vi "Get Buffer Data from Variant.vi"(8 "error in (no error)":errorcluster, 10 "tag":string, 11 "Application Data In in":T2) -> (0 "error out":errorcluster, 1 "Buffer data":T1 {"avg bandwidth" format="%.0g bytes"}, 3 "Application Data In out":T2)   [LabVIEW 2017, in "DSF Core.lvlib"]
uses:
  DSF Core.lvlib
  Main VI/Application Data.ctl
  <vilib>/NI/Memory Manager/Classes/Pointer/Pointer.lvclass
  Classes/Framework/Framework.lvclass
  Buffer Reader/Buffer Data.ctl
  Classes/Buffer/Buffer.lvclass
  Classes/Transfer Group Status/Transfer Group Status.lvclass
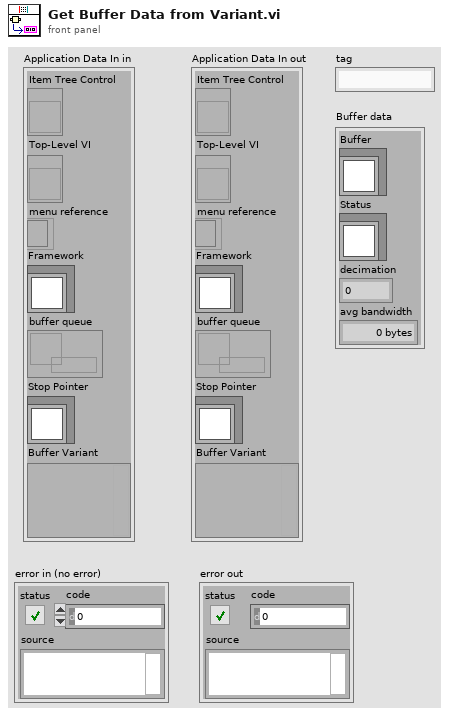
[diagram p1: front panel]
types:
  T1 = typedef "DSF Core.lvlib/Buffer Data.ctl" = cluster{"Buffer":refnum<class "Buffer.lvclass">, "Status":refnum<class "Transfer Group Status.lvclass">, "decimation":u64, "avg bandwidth":dbl}
  T2 = typedef "DSF Core.lvlib/Application Data.ctl" = cluster{"Item Tree Control":refnum<vi>, "Top-Level VI":refnum<vi>, "menu reference":refnum<k9>, "Framework":refnum<class "Framework.lvclass">, "buffer queue":refnum<queue>, "Stop Pointer":refnum<class "Pointer.lvclass">, "Buffer Variant":variant}
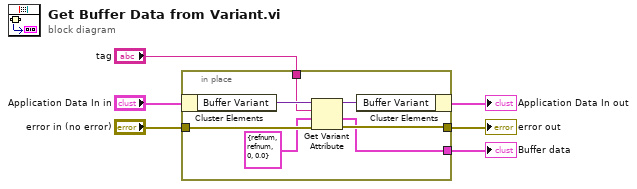
[diagram p0: block diagram]
diagram:
  n1 = in-place {
    in-place-border: [w11] -> w3
    in-place-border: "error in (no error)" -> [w12]
    in-place-border: "tag" -> [w10]
    in-place-border: [w7] -> w1
    n2 = in-place-cluster #1("Application Data In in") -> ("Buffer Variant"=w13:variant)
    n3 = Get Variant Attribute(Variant=w13, name=w10, default value (empty Variant)=T1 {"Buffer"=refnum, "Status"=refnum, "decimation"=0, "avg bandwidth"=0.0} ("Buffer data"), error in=w12) -> (duplicate Variant=w9:variant, value=w7:T1, error out=w11:errorcluster)  [unwired: 1 out]
    n4 = in-place-cluster #1("Buffer Variant"=w9) -> (→"Application Data In out":T2)
  }
  "error out" <- w3
  "Buffer data" <- w1
